vi "SetDialogBoxesToModal.vi"(8 "ErrorIn":errorcluster) -> (0 "ErrorOut":errorcluster)   [LabVIEW 2018]
doc: "For Development System mode, force all of the VIs within the DialogBoxes folder to be set to Modal.\n\nThis is useful during development to guarantee that there is only one active window. \n\nUse with caution, because it overrides any non-modal (default) or floating settings that windows may have, so don't use this if you need any non-modal windows.\n\nKillAllModals.vi can be used to kill any VIs that have been forced into modal mode with this VI.\n\nCopyright © 2019 Epimedia, Inc. All Rights Reserved.\n\nThe Epimedia Application Library is Copyright © 2009-2017 Epimedia, Inc. \nAll Rights Reserved. Used under license."
panel:
  # "Copyright © 2019 Epimedia, Inc. All Rights Reserved.\n\nThe Epimedia Application Library is Copyright © 2009-2017 Epimedia, Inc. \nAll Rights Reserved. Used under license."
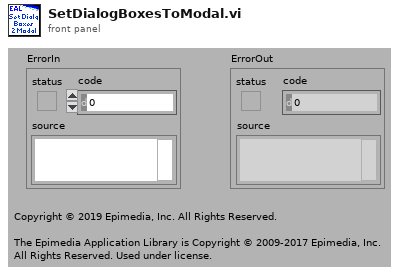
[diagram p1: front panel]
types:
  T1 = enum32{"invalid app kind", "Development System", "Run Time System", "Student Edition", "Embedded LabVIEW", "Evaluation", "Custom"}
  T2 = enum32{"Invalid", "Default", "Floating", "Floating/Auto-Hide", "Modal"}
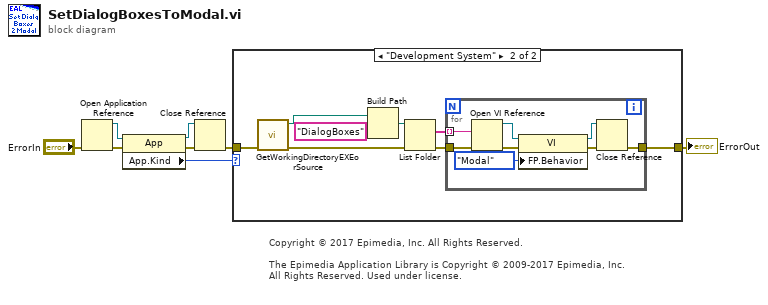
[diagram p0: block diagram]
diagram:
  # "Copyright © 2017 Epimedia, Inc. All Rights Reserved.\n\nThe Epimedia Application Library is Copyright © 2009-2017 Epimedia, Inc. \nAll Rights Reserved. Used under license."
  n1 = Open Application Reference(8:"ErrorIn") -> (0:w7:errorcluster, 3:w6:refnum<vi>)  [unwired: 3 in]
  n2 = property class="App"(reference=w6, error in=w7) -> (reference out=w3:refnum<vi>, error out=w2:errorcluster, "App.Kind"=w5:T1)
  n3 = Close Reference(reference=w3, error in (no error)=w2) -> (error out=w1:errorcluster)
  n4 = case shown="\"Development System\"" w5 {
    tunnel: w1 -> [w9 w11]
    tunnel: [w9 w10] -> w4
    frame Default {
    }
    frame "Development System" {
      n5 = call "GetWorkingDirectoryEXEorSource.vi"("ErrorIn"=w11) -> ("ErrorOut"=w14:errorcluster, "Directory"=w17:path)  [unwired: 9 in]
      n6 = Build Path(base path=w17, name or relative path="DialogBoxes") -> (appended path=w15:path)
      n7 = List Folder(path=w15, error in=w14) -> (filenames=w12:string[], error out=w13:errorcluster)  [unwired: 2 in, 2 out]
      n8 = for {
        tunnel: w12 -> [w24] mode=indexing
        tunnel: w13 -> [w25]
        tunnel: [w21] -> w10
        n9 = Open VI Reference(vi path=w24, error in (no error)=w25) -> (vi reference=w19:refnum<vi>, error out=w18:errorcluster)  [unwired: 4 in]
        n10 = property class="VI"(reference=w19, error in=w18, "FP.Behavior"=T2."Modal" ("Front Panel Window:Behavior")) -> (reference out=w22:refnum<vi>, error out=w23:errorcluster)
        n11 = Close Reference(reference=w22, error in (no error)=w23) -> (error out=w21:errorcluster)
      }
    }
  }
  "ErrorOut" <- w4
